vi "Inventario Path--constant.vi"() -> (3 "Ruta Inventario":path)   [LabVIEW 2024, in "ProductControl.lvlib"]
uses:
  ProductControl.lvlib
panel:
  out "Ruta Inventario EXE":path
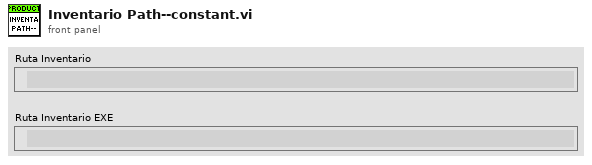
[diagram p1: front panel]
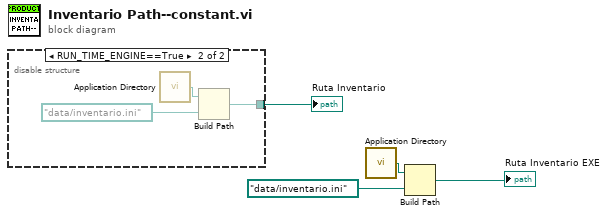
[diagram p0: block diagram]
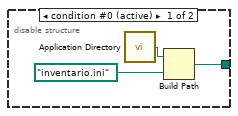
[diagram p2: hidden frame]
diagram:
  n1 = disable-structure shown="RUN_TIME_ENGINE==True" {
    disable-tunnel: [w7 w10] -> w4
    frame condition #0 (active) {
      n2 = call <vilib>:"Application Directory.vi"() -> ("Application Directory"=w5:path)
      n3 = Build Path(base path=w5, name or relative path=path "inventario.ini") -> (appended path=w7:path)
    }
    frame condition #1 {
      n4 = call <vilib>:"Application Directory.vi"() -> ("Application Directory"=w8:path)
      n5 = Build Path(base path=w8, name or relative path=path "data/inventario.ini") -> (appended path=w10:path)
    }
  }
  "Ruta Inventario" <- w4
  n6 = call <vilib>:"Application Directory.vi"() -> ("Application Directory"=w3:path)
  n7 = Build Path(base path=w3, name or relative path=path "data/inventario.ini") -> (appended path=→"Ruta Inventario EXE":path)
